vi "Main RT.vi"() -> ()   [LabVIEW 2019]
uses:
  <vilib>/Platform/TimedLoop/XDataNode/timing_clust.ctl
  <vilib>/Platform/TimedLoop/XDataNode/nitl_modes.ctl
  <vilib>/Platform/TimedLoop/XDataNode/wakeup.ctl
  <vilib>/FPGAPlugInAG/myRIO-1900/niLvFpga_Open_myRIO-1900.vi
  <vilib>/rvi/interface/common/dynamic/niFpgaDynamicAddResources.vi
  <vilib>/Utility/error.llb/Error Cluster From Error Code.vi
  <vilib>/rvi/errors/niLvFpgaAdjustHostInterfaceError.vi
  <vilib>/FPGAPlugInAG/Dynamic/niLvFpga_Close_Dynamic.vi
  <vilib>/rvi/interface/nirviOpenFPGA/nirviOpenFPGA.xnode
  FPGA Bitfiles/ledmatrix_FPGATarget_MainFPGA_p8SXomXGKcI.lvbitx
  <vilib>/rvi/interface/nirviReadWriteControl/nirviReadWriteControl.xnode
  <vilib>/rvi/interface/nirviCloseFPGA/nirviCloseFPGA.xnode
  <vilib>/Platform/TimedLoop/XDataNode/XDataNode.xnode
  <vilib>/rvi/interface/nirviMethod/nirviMethod.xnode
  <vilib>/Platform/TimedLoop/XDataNode/XDNodeRunTimeDep.lvlib
  <vilib>/FPGAPlugInAG/Dynamic/niLvFpga_ReadFifo_Dynamic.vi
  <vilib>/rvi/errors/niLvFpgaMergeErrorWithErrorCode.vi
  NiFpgaLv.dll
  <vilib>/rvi/interface/Simulation/niFpgaSimulationCallBeginRW.vi
panel:
  out "Array":cluster{u32, bool}[](array[cluster])
  out "interleaved array":u8[](array[numeric])
  in  "B":sgl(slide) scale=0.0..1.0
  in  "G":sgl(slide) scale=0.0..1.0
  in  "R":sgl(slide) scale=0.0..1.0
  out "Waveform Graph":waveform(dbl)(graph)
  in  "Intensity":sgl(slide) scale=0.0..1.0
  out "Data":bool[](array[boolean])
  in  "Reset":u16=2000
  in  "Low False":u16=600
  in  "Low True":u16=300
  in  "High False":u16=300
  in  "High True":u16=600
  in  "stop":bool
  out "Timed Out?":bool
  in  "Update":bool
  # "1536 bits per frame"
  # "1843us takes the whole frame"
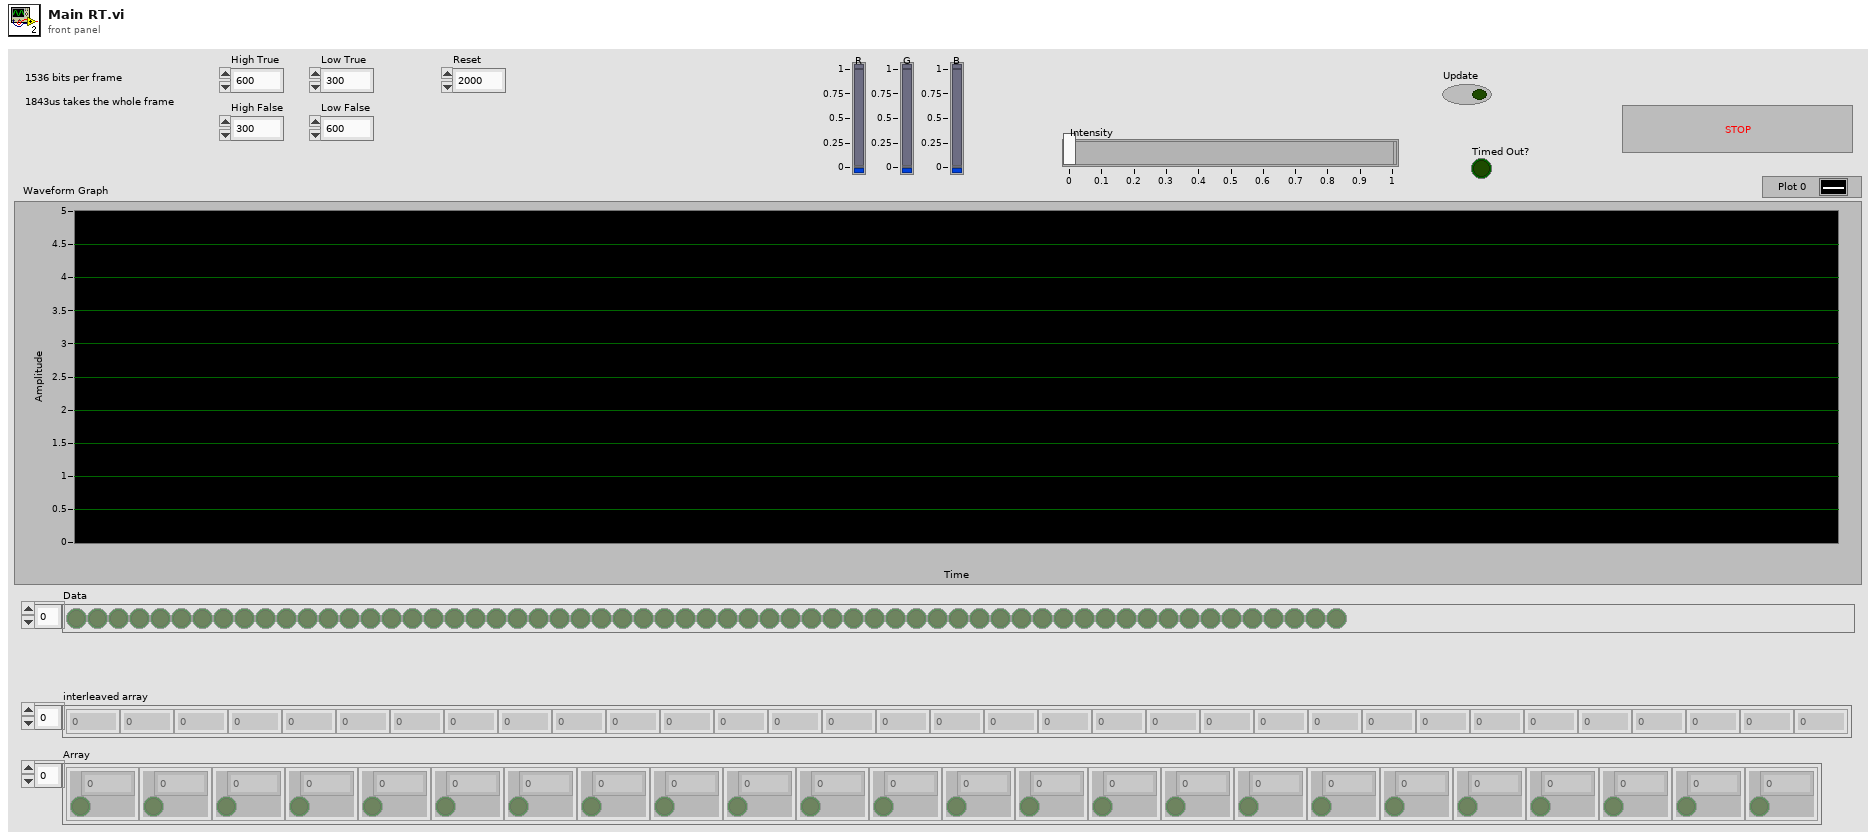
[diagram p1: front panel]
types:
  T1 = typedef "XDNodeRunTimeDep.lvlib/timing_clust.ctl" = cluster{"Expected End [f-1]":u64, "Actual End [f-1]":u64, "Finished Late? [f-1]":bool, "Expected End [i-1]":u64, "Actual End [i-1]":u64, "Finished Late? [i-1]":bool, "Expected Start [i]":u64, "Actual Start [i]":u64, "Expected Start [f]":u64, "Actual Start [f]":u64, "Source Name":string, "Structure Name":string, "Period":i64, "Deadline":i64, "Offset":i64, "Start":i64, "Priority":i32, "Timeout":i32, "Mode":T2, "Wakeup Reason":T3, "Error":errorcluster, "Source Type":string, "Secondary Source Type":string, "Global End Time":u64, "Global Start Time":u64, "Frame Duration":u64, "Iteration Duration":u64, "Assigned CPU":i32, "I/O Scan Engine Mode":u32}
  T2 = typedef "XDNodeRunTimeDep.lvlib/nitl_modes.ctl" = enum32{"No Change", "Process missed periods, maintain original phase", "Discard missed periods, maintain original phase", "Process missed periods, ignore original phase", "Discard missed periods, ignore original phase"}
  T3 = typedef "XDNodeRunTimeDep.lvlib/wakeup.ctl" = enum32{"Normal", "Aborted", "Asynchronous wakeup", "Timing source error", "Timed loop error", "Timeout"}
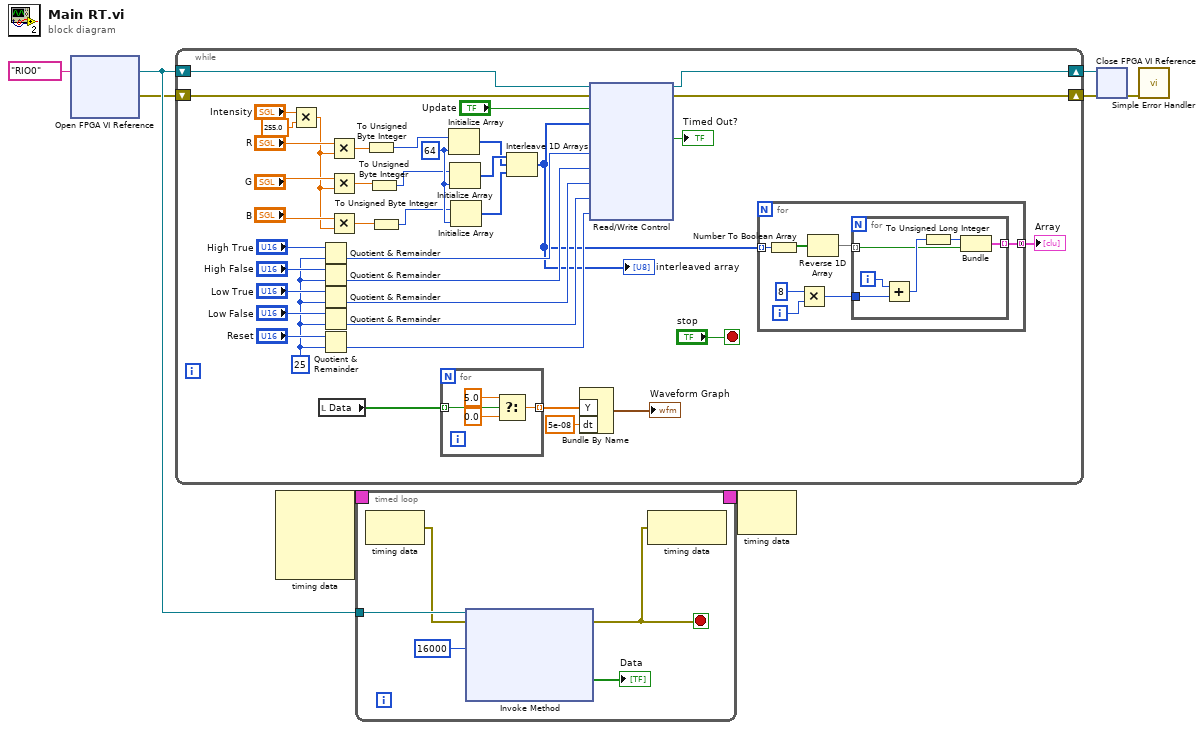
[diagram p0: block diagram]
diagram:
  n1 = xnode "Open FPGA VI Reference"("resource name"=tag "RIO0") -> ("FPGA VI Reference Out"=w5:refnum<k20>, "error out"=w1:errorcluster)  [unwired: 1 in]
  n2 = while {
    shift-right: [w44] -> w7
    shift-left: w5 -> [w48]
    shift-right: [w43] -> w6
    shift-left: w1 -> [w47]
    stop <- "stop" stop-if-true
    w32 = u16 25 ("y")
    w40 = 64 ("dimension size")
    n3 = Multiply(x="Intensity", y=sgl 255.0) -> (x*y=w18:sgl)
    n4 = local read "Data"() -> (w26:bool[])
    n5 = Quotient & Remainder(x="High True", y=w32) -> (floor(x/y)=w31:u16)  [unwired: 1 out]
    n6 = Quotient & Remainder(x="High False", y=w32) -> (floor(x/y)=w30:u16)  [unwired: 1 out]
    n7 = Quotient & Remainder(x="Low True", y=w32) -> (floor(x/y)=w29:u16)  [unwired: 1 out]
    n8 = Quotient & Remainder(x="Low False", y=w32) -> (floor(x/y)=w28:u16)  [unwired: 1 out]
    n9 = Quotient & Remainder(x="Reset", y=w32) -> (floor(x/y)=w27:u16)  [unwired: 1 out]
    n10 = Multiply(x="R", y=w18) -> (x*y=w14:sgl)
    n11 = Multiply(x="G", y=w18) -> (x*y=w16:sgl)
    n12 = Multiply(x="B", y=w18) -> (x*y=w15:sgl)
    n13 = To Unsigned Byte Integer(number=w14) -> (unsigned 8bit integer=w13:u8)
    n14 = To Unsigned Byte Integer(number=w16) -> (unsigned 8bit integer=w12:u8)
    n15 = To Unsigned Byte Integer(number=w15) -> (unsigned 8bit integer=w11:u8)
    n16 = for {
      tunnel: [w63] -> w22 mode=indexing
      tunnel: w26 -> [w62] mode=indexing
      n17 = Select(t=5.0, s=w62, f=0.0) -> (s? t:f=w63:dbl)
    }
    n18 = Initialize Array(w13, w40) -> (w38:u8[])
    n19 = Initialize Array(w12, w40) -> (w39:u8[])
    n20 = Initialize Array(w11, w40) -> (w41:u8[])
    n21 = Interleave 1D Arrays(w39, w38, w41) -> (w10:u8[])
    "interleaved array" <- w10
    n22 = Bundle By Name("Y"=w22, "dt"=5e-08) -> (→"Waveform Graph":waveform(dbl))  [unwired: 1 in]
    n23 = xnode "Read/Write Control"("FPGA VI Reference In"=w48, "error in"=w47, "Update"="Update", "Matrix Array"=w10, "High True"=w31, "High False"=w30, "Low True"=w29, "Low False"=w28, "Reset (us)"=w27) -> ("FPGA VI Reference Out"=w44:refnum<k20>, "error out"=w43:errorcluster, "Timed Out?"=→"Timed Out?":bool)
    n24 = for {
      tunnel: w10 -> [w52] mode=indexing
      tunnel: [w51] -> w9 mode=concatenating
      i -> [w55]
      n25 = Number To Boolean Array(number=w52) -> (Boolean array=w49:bool[])
      n26 = Multiply(x=8, y=w55) -> (x*y=w53:i32)
      n27 = Reverse 1D Array(array=w49) -> (reversed array=w50:bool[])
      n28 = for {
        tunnel: w50 -> [w57] mode=indexing
        tunnel: w53 -> [w60]
        tunnel: [w56] -> w51 mode=indexing
        i -> [w61]
        n29 = Add(x=w61, y=w60) -> (x+y=w59:i32)
        n30 = To Unsigned Long Integer(number=w59) -> (unsigned 32bit integer=w58:u32)
        n31 = Bundle(w58, w57) -> (w56:cluster{u32, bool})  [unwired: 1 in]
      }
    }
    "Array" <- w9
  }
  n32 = node-c288() -> (w4:T1)  [unwired: 4 in]
  n33 = timed-loop {
    timing: w4 -> [_]
    timing-out: [_] -> w3
    tunnel: w5 -> [w70]
    stop <- w66 stop-if-true
    n34 = node-c288() -> (w67:errorcluster)  [unwired: 1 in]
    n35 = xnode "Invoke Method"("FPGA VI Reference In"=w70, "error in"=w67, "Number of Elements"=u32 16000) -> ("error out"=w66:errorcluster, "Data"=→"Data":bool[])  [unwired: 1 in, 2 out]
    n36 = node-c288(w66) -> ()  [unwired: 1 out]
  }
  n37 = node-c288(w3) -> ()  [unwired: 1 out]
  n38 = xnode "Close FPGA VI Reference"("FPGA VI Reference In"=w7, "error in"=w6) -> ("error out"=w2:errorcluster)
  n39 = call <vilib>:"Simple Error Handler.vi"("error in (no error)"=w2) -> ()  [unwired: 4 in, 5 out]
